vi "mark values RL AF CP.vi"(4 "AF loc. index":i32, 6 "Contact Point index":i32, 7 "RL index":i32, 9 "X":dbl[](array[numeric]), 10 "Y":dbl[](array[numeric]), 11 "XYGraph in":refnum<vi>) -> ()   [LabVIEW 2015]
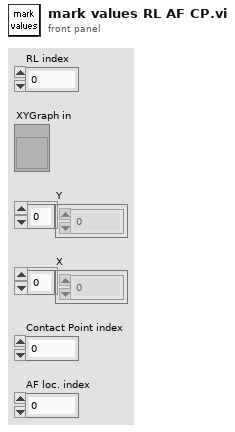
[diagram p1: front panel]
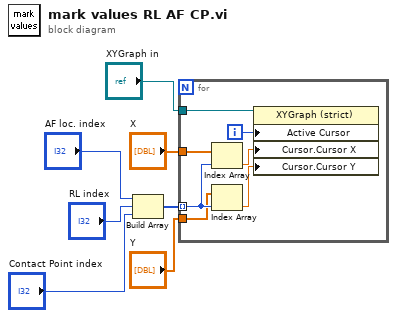
[diagram p0: block diagram]
diagram:
  n1 = Build Array("AF loc. index", "RL index", "Contact Point index") -> (w5:i32[])
  n2 = for {
    tunnel: "XYGraph in" -> [w14]
    tunnel: w5 -> [w12] mode=indexing
    tunnel: "X" -> [w11]
    tunnel: "Y" -> [w10]
    i -> [w13]
    n3 = Index Array(array=w11, index=w12) -> (element=w9:dbl)
    n4 = Index Array(array=w10, index=w12) -> (element=w8:dbl)
    n5 = property class="XYGraph (strict)"(reference=w14, "Active Cursor"=w13, "Cursor.Cursor X"=w9, "Cursor.Cursor Y"=w8) -> ()  [unwired: 1 in, 2 out]
  }
